vi "Arduino Write Bytes.vi"(8 "error in (no error)":errorcluster, 9 "Bytes":u8[](array[numeric]), 10 "Command":string, 11 "COM Port In":refnum<visa-resource-name>) -> (0 "error out":errorcluster, 1 "OK?":bool, 2 "Response":string, 3 "COM Port Out":refnum<visa-resource-name>)   [LabVIEW 2023, in "Arduino DAQ.lvlib"]
uses:
  Arduino DAQ.lvlib
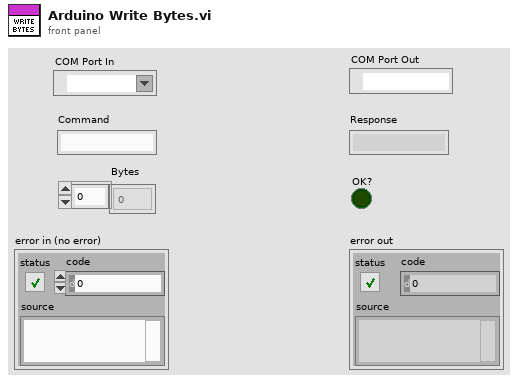
[diagram p1: front panel]
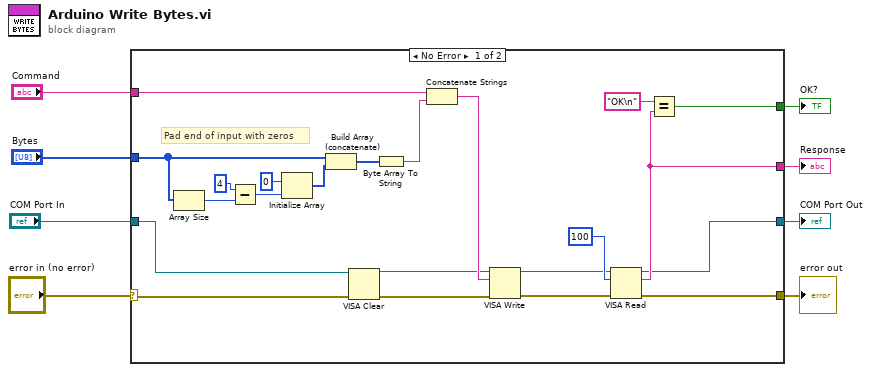
[diagram p0: block diagram]
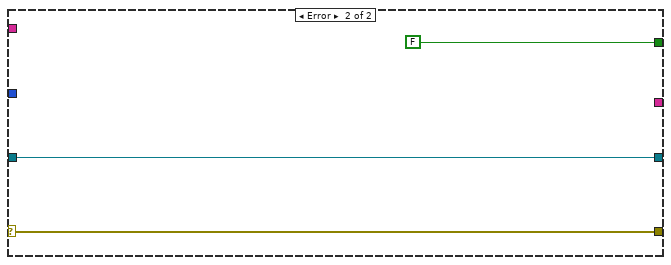
[diagram p2: hidden frame]
diagram:
  n1 = case shown="No Error" "error in (no error)" {
    selector: "error in (no error)" -> [w9 w33]
    tunnel: [w28 w33] -> w8
    tunnel: "COM Port In" -> [w10 w31]
    tunnel: [w27 _] -> w5
    tunnel: [w25 FALSE] -> w4
    tunnel: "Command" -> [w23 _]
    tunnel: "Bytes" -> [w19 _]
    tunnel: [w13 w31] -> w1
    frame No Error {
      # "Pad end of input with zeros"
      n2 = Array Size(array=w19) -> (size(s)=w21:i32)
      n3 = Subtract(x=4, y=w21) -> (x-y=w17:i32)
      n4 = Initialize Array(u8 0 ("element"), w17) -> (w18:u8[])
      n5 = Build Array (concatenate)(w19, w18) -> (w15:u8[])
      n6 = VISA Clear(VISA resource name=w10, error in (no error)=w9) -> (VISA resource name out=w11:refnum<visa-resource-name>, error out=w12:errorcluster)
      n7 = Byte Array To String(unsigned byte array=w15) -> (string=w14:string)
      n8 = Concatenate Strings(w23, w14) -> (w22:string)
      n9 = VISA Write(VISA resource name=w11, write buffer=w22, error in (no error)=w12) -> (VISA resource name out=w24:refnum<visa-resource-name>, error out=w29:errorcluster)  [unwired: 1 out]
      n10 = VISA Read(VISA resource name=w24, byte count=u32 100, error in (no error)=w29) -> (VISA resource name out=w13:refnum<visa-resource-name>, read buffer=w27:string, error out=w28:errorcluster)  [unwired: 1 out]
      n11 = Equal?(x="OK\n" ("y"), y=w27) -> (x = y?=w25:bool)
    }
    frame Error {
    }
  }
  "Response" <- w5
  "OK?" <- w4
  "error out" <- w8
  "COM Port Out" <- w1
